vi "New BetterListboxHandle.vi"(8 "error in (no error)":errorcluster, 10 "TreeBar Picture Ref":refnum<vi>, 11 "LB ref":refnum<vi>) -> (0 "error out":errorcluster, 3 "BetterListboxHandle out":refnum<class "BetterListboxHandle.lvclass">)   [LabVIEW 2020, in "BetterDragAndDrop.lvlib" / "BetterListboxHandle.lvclass"]
uses:
  BetterListboxHandle.lvclass
  C:/DSCE code/Open-source/betterdraganddrop_GIT/Source/Classes/BetterHandle/BetterHandle.lvclass
  BetterListboxHandle.lvclass/BetterListboxHandle.ctl
  BetterHandle/BetterHandle.lvclass/BetterHandle.ctl
  BetterHandle/Write TreeBar.vi
  BetterTreeBar/BetterHorizontalBar.lvclass
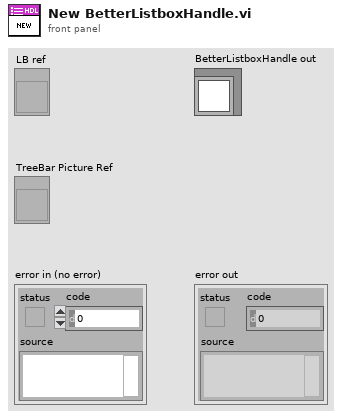
[diagram p1: front panel]
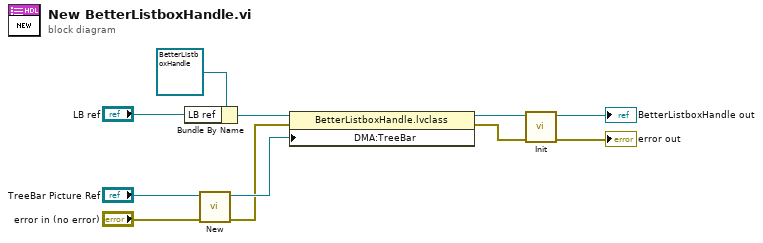
[diagram p0: block diagram]
diagram:
  n1 = Bundle By Name(cluster=refnum<class "BetterListboxHandle.lvclass"> refnum ("BetterListboxHandle out"), "LB ref"="LB ref") -> (w7:refnum<class "BetterListboxHandle.lvclass">)
  n2 = call "New.vi"("error in (no error)"="error in (no error)", "Picture Ref"="TreeBar Picture Ref") -> ("error out"=w3:errorcluster, "BetterTreeBar out"=w6:refnum<class "BetterHorizontalBar.lvclass">)  [unwired: 8 in]
  n3 = property class="BetterListboxHandle.lvclass"(reference=w7, error in=w3, "DMA:TreeBar"=w6) -> (reference out=w5:refnum<class "BetterListboxHandle.lvclass">, error out=w2:errorcluster)
  n4 = call-dynamic "Init.vi"("error in (no error)"=w2, "BetterListboxHandle in"=w5) -> ("error out"=→"error out":errorcluster, "BetterListboxHandle out"=→"BetterListboxHandle out":refnum<class "BetterListboxHandle.lvclass">)  [unwired: 8 in]
